vi "Do.vi"(8 "error in":errorcluster, 10 "Actor in":refnum<class "Actor.lvclass">, 11 "Send New Setpoint":refnum<class "Send New Setpoint.lvclass">) -> (0 "error out":errorcluster, 2 "Actor out":refnum<class "Actor.lvclass">)   [LabVIEW 2014, in "Device.lvlib" / "Send New Setpoint.lvclass"]
doc: "(<B>Filename</B>: Actor Framework.lvlib:Message.lvclass:Do.vi)\n\nDefines what a message does when it is received by an actor. Generally, a message instructs an actor to invoke one of its methods. By default, this method does nothing. A child class must override it to define behavior. Create a child class by using the Actor Framework Message Maker dialog box."
uses:
  Send New Setpoint.lvclass
  <vilib>/ActorFramework/Actor/Actor.lvclass
  Send New Setpoint.lvclass/Send New Setpoint.ctl
  reusable/DAQ Device/Device/Device.lvclass
  reusable/DAQ Device/Device/Device.lvclass/Device.ctl
  reusable/DAQ Device/Device/Read Configurable Device.vi
  Configurable Device.lvclass
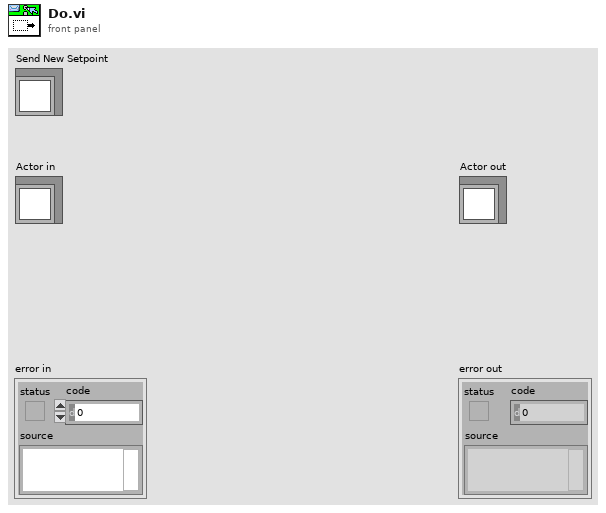
[diagram p1: front panel]
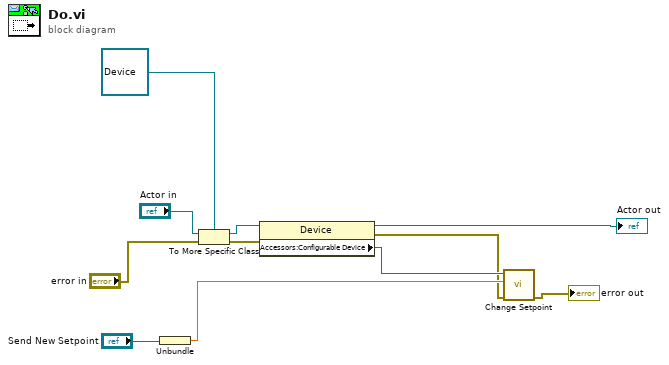
[diagram p0: block diagram]
diagram:
  n1 = Unbundle("Send New Setpoint") -> (w3:dbl)
  n2 = To More Specific Class(target class=refnum<class "Device.lvclass"> refnum ("DAQ Device.lvlib:Device"), reference="Actor in", error in="error in") -> (specific class reference=w8:refnum<class "Device.lvclass">, error out=w7:errorcluster)
  n3 = property class="Device"(reference=w8, error in=w7) -> (reference out=→"Actor out":refnum<class "Device.lvclass">, error out=w2:errorcluster, "Accessors:Configurable Device"=w4:refnum<class "Configurable Device.lvclass">)
  n4 = call-dynamic "Change Setpoint.vi"("error in (no error)"=w2, "Setpoint"=w3, "Configurable Device in"=w4) -> ("error out"=→"error out":errorcluster)  [unwired: 7 in, 1 out]
